vi "Read msn.vi"(8 "error in (no error)":errorcluster, 11 "MessagE in":refnum<class "Message.lvclass">) -> (0 "error out":errorcluster, 3 "MessagE out":refnum<class "Message.lvclass">)   [LabVIEW 2021, in "Msn Trasnsportation Library 1.lvlib" / "Message.lvclass"]
uses:
  Message.lvclass
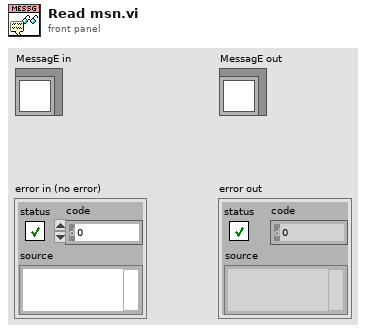
[diagram p1: front panel]
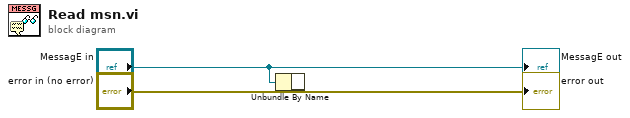
[diagram p0: block diagram]
diagram:
  n1 = Unbundle By Name("MessagE in") -> ()  [unwired: 1 out]
  "error out" <- "error in (no error)"
  "MessagE out" <- "MessagE in"
